vi "Write Number of channels.vi"(10 "Number of channels":i8=1, 11 "Oscilloscope in":refnum<class "Oscilloscope.lvclass">) -> (3 "Oscilloscope out":refnum<class "Oscilloscope.lvclass">)   [LabVIEW 2020, in "Oscilloscope.lvclass"]
uses:
  Oscilloscope.lvclass
  Oscilloscope.lvclass/Oscilloscope.ctl
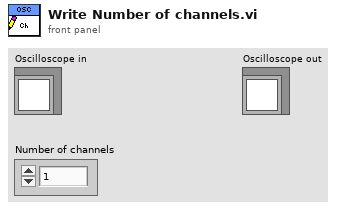
[diagram p1: front panel]
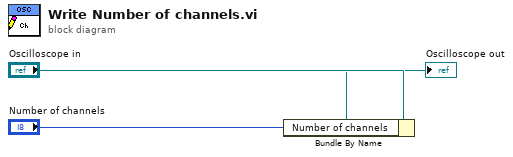
[diagram p0: block diagram]
diagram:
  n1 = Bundle By Name(cluster="Oscilloscope in", "Number of channels"="Number of channels") -> (→"Oscilloscope out":refnum<class "Oscilloscope.lvclass">)
